vi "flat top.vi"() -> ()   [LabVIEW 2016]
doc: "takes a given beamline component and steps through values and reocrnds the current\noutput from a faraday cup. Allows user to pick highest value"
uses:
  Main/beamline selection.ctl
  Controls/Flat top control settings.ctl
  Controls/flat top states.ctl
  Beamline sections/Main VIs/LowEnd.vi
  Top level/flat top/flat top.lvlib
  Main/main.lvlib
  Beamline sections/Low Energy End/Low energy.lvlib
panel:
  in  "Tab Control":enum32{"Flat Top", "Info", "Errors"}(tab)
  out "Flat top results":cluster{"Y":dbl[], "Y":dbl[]}[](graph)
  in  "Control items":u16(ring) items=["Injector Image X steerer", "Injector Image Y steerer ", "Low Energy Waist  X steerer", "Low Energy Waist Y steerer ", "Tank Entrance  X steerer ", "Tank Entrance Y1 steerer ", "Tank Entrance Y2 steerer ", "Injector Image Einzel ", "Low Energy Einzel ", "Low Energy Waist aperture"]
  in  "Beamline Section":T1
  in  "Flat Top Control Settings":T2={"Start value"=0.0, "Number of steps"=100.0, "Ramp Up Time (s)"=0.0, "End value"=1.0, "Integration Time (s)"=15.0}
  out "step size":dbl
  in  "rare or stable":bool=TRUE
  out "Method of flat top":string
  in  "flat top":bool
  in  "stop":bool
  in  "Help":bool
  out "Main Loop Error":bool=TRUE
  out "Step":i32
  in  "Clear FT Loop Errors":bool
  in  "Clear Main Loop Errors":bool
  out "Main loop error":errorcluster
  out "Flat Top loop error":errorcluster
  out "Original Setting":dbl
  in  "?":cluster{"X":dbl[], "Y":dbl[]}
  in  "error in (no error)":errorcluster
  # "Rare count rate"
  # "Stable Current"
  # "Instructions\n\n1. \n2. \n3."
  # "Notes\n\nPausing/Re-starting\n\nStopping"
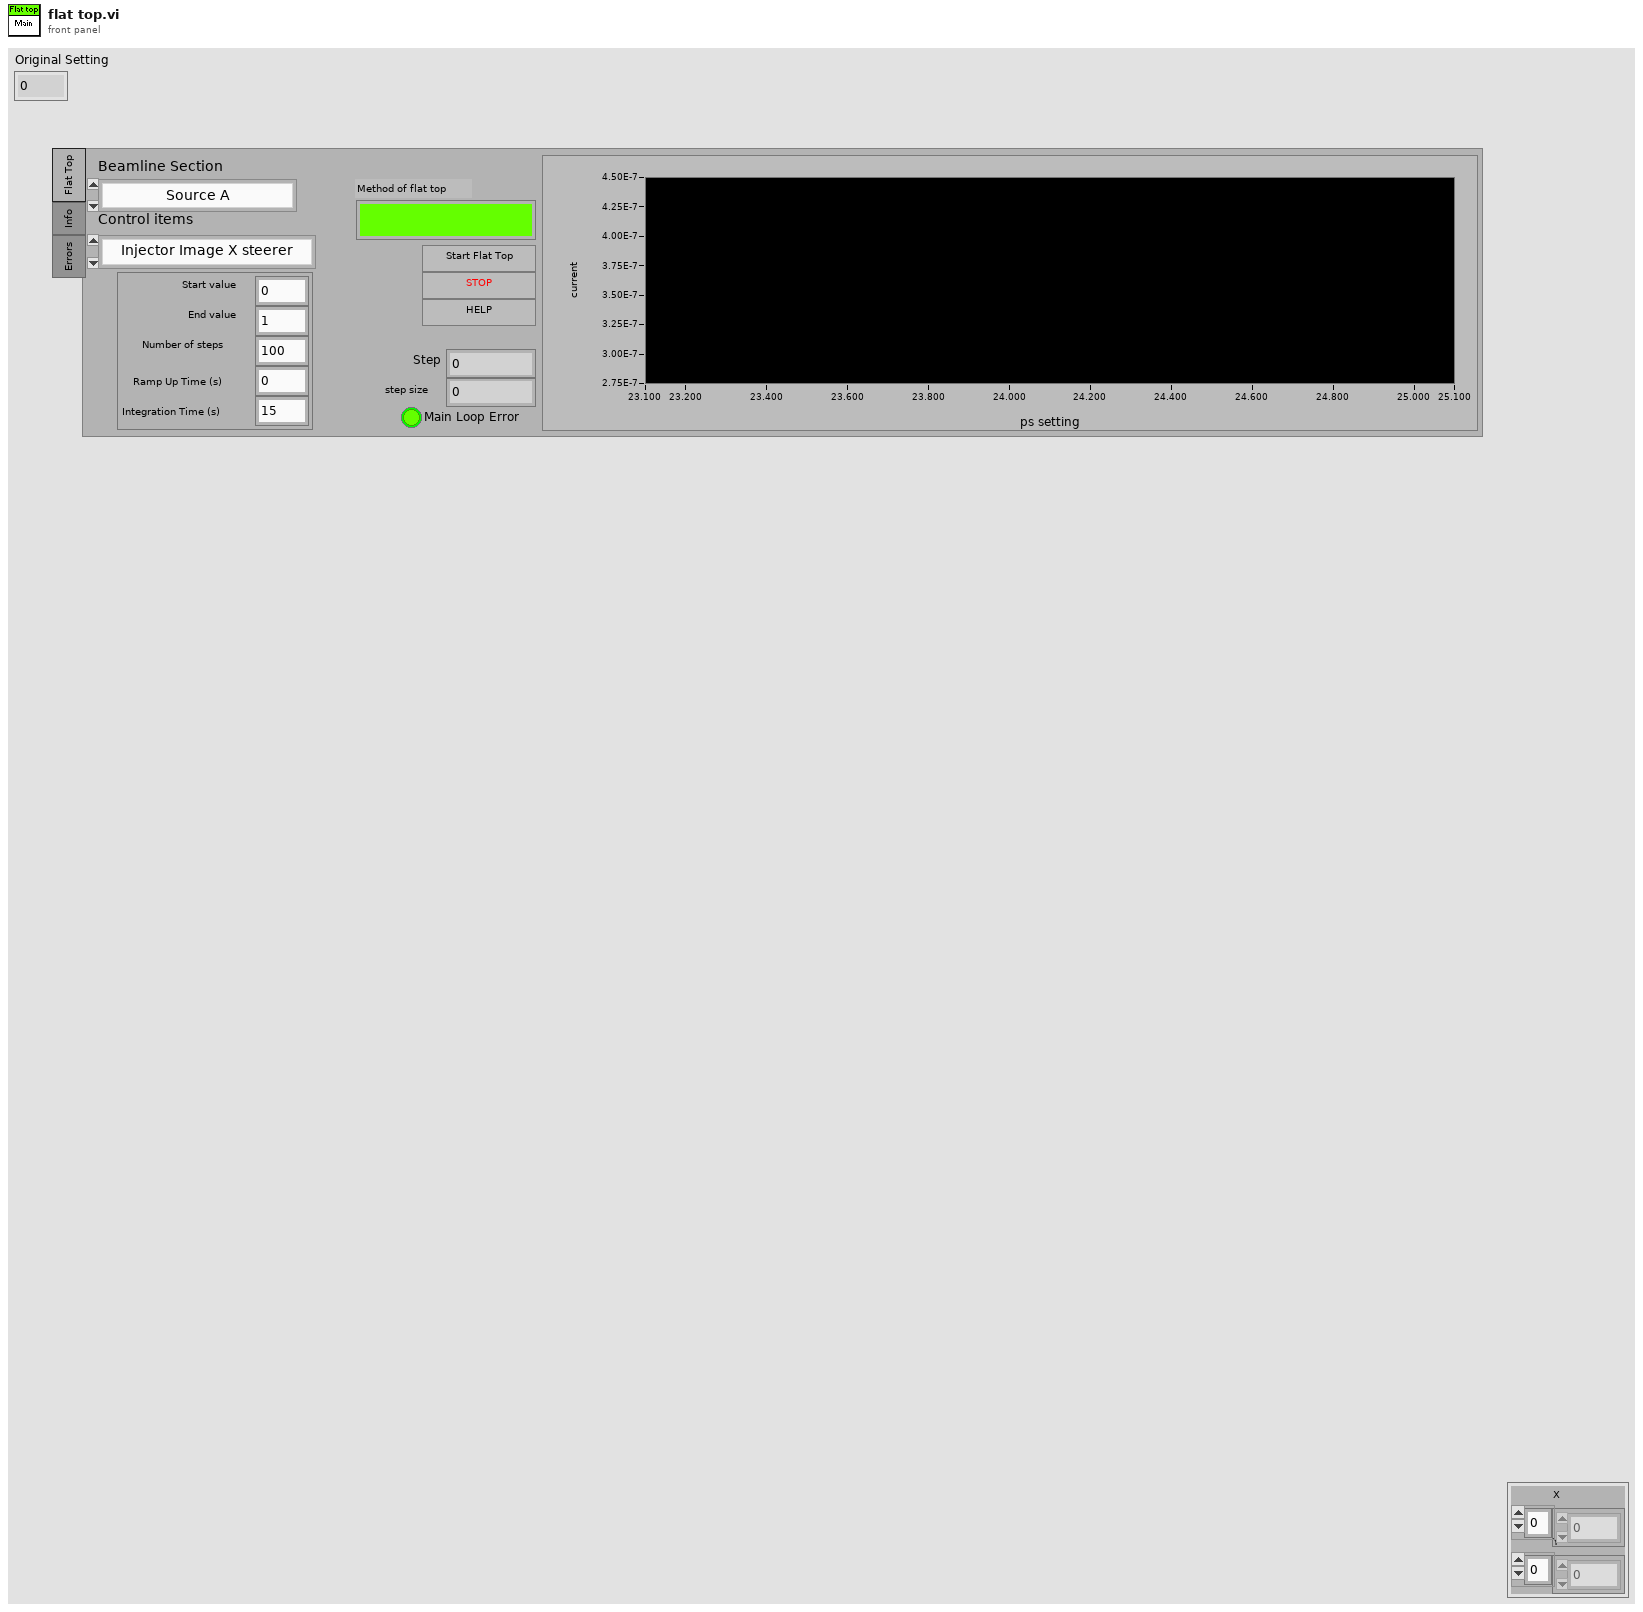
[diagram p1: front panel]
types:
  T1 = typedef "main.lvlib/beamline selection.ctl" = enum16{"Source A", "Low End", "High End", "Transmission", "R30", "R45"}
  T2 = typedef "Flat top control settings.ctl" = cluster{"Start value":dbl, "Number of steps":dbl, "Ramp Up Time (s)":dbl, "End value":dbl, "Integration Time (s)":dbl}
  T3 = typedef "flat top states.ctl" = enum16{"wait", "pause", "flat top", "stop"}
  T4 = cluster{"beamline name":string, "inital value":dbl}[]
  T5 = enum8{"Enabled", "Disabled", "Disabled and Grayed Out"}
  T6 = cluster{"beamline name":string, "inital value":dbl}
  T7 = typedef "LVPoint32TypeDef.ctl" = cluster{"Horizontal":i32, "Vertical":i32}
  T8 = enum16{"Left Button", "Center Button", "Right Button", "Window Close"}
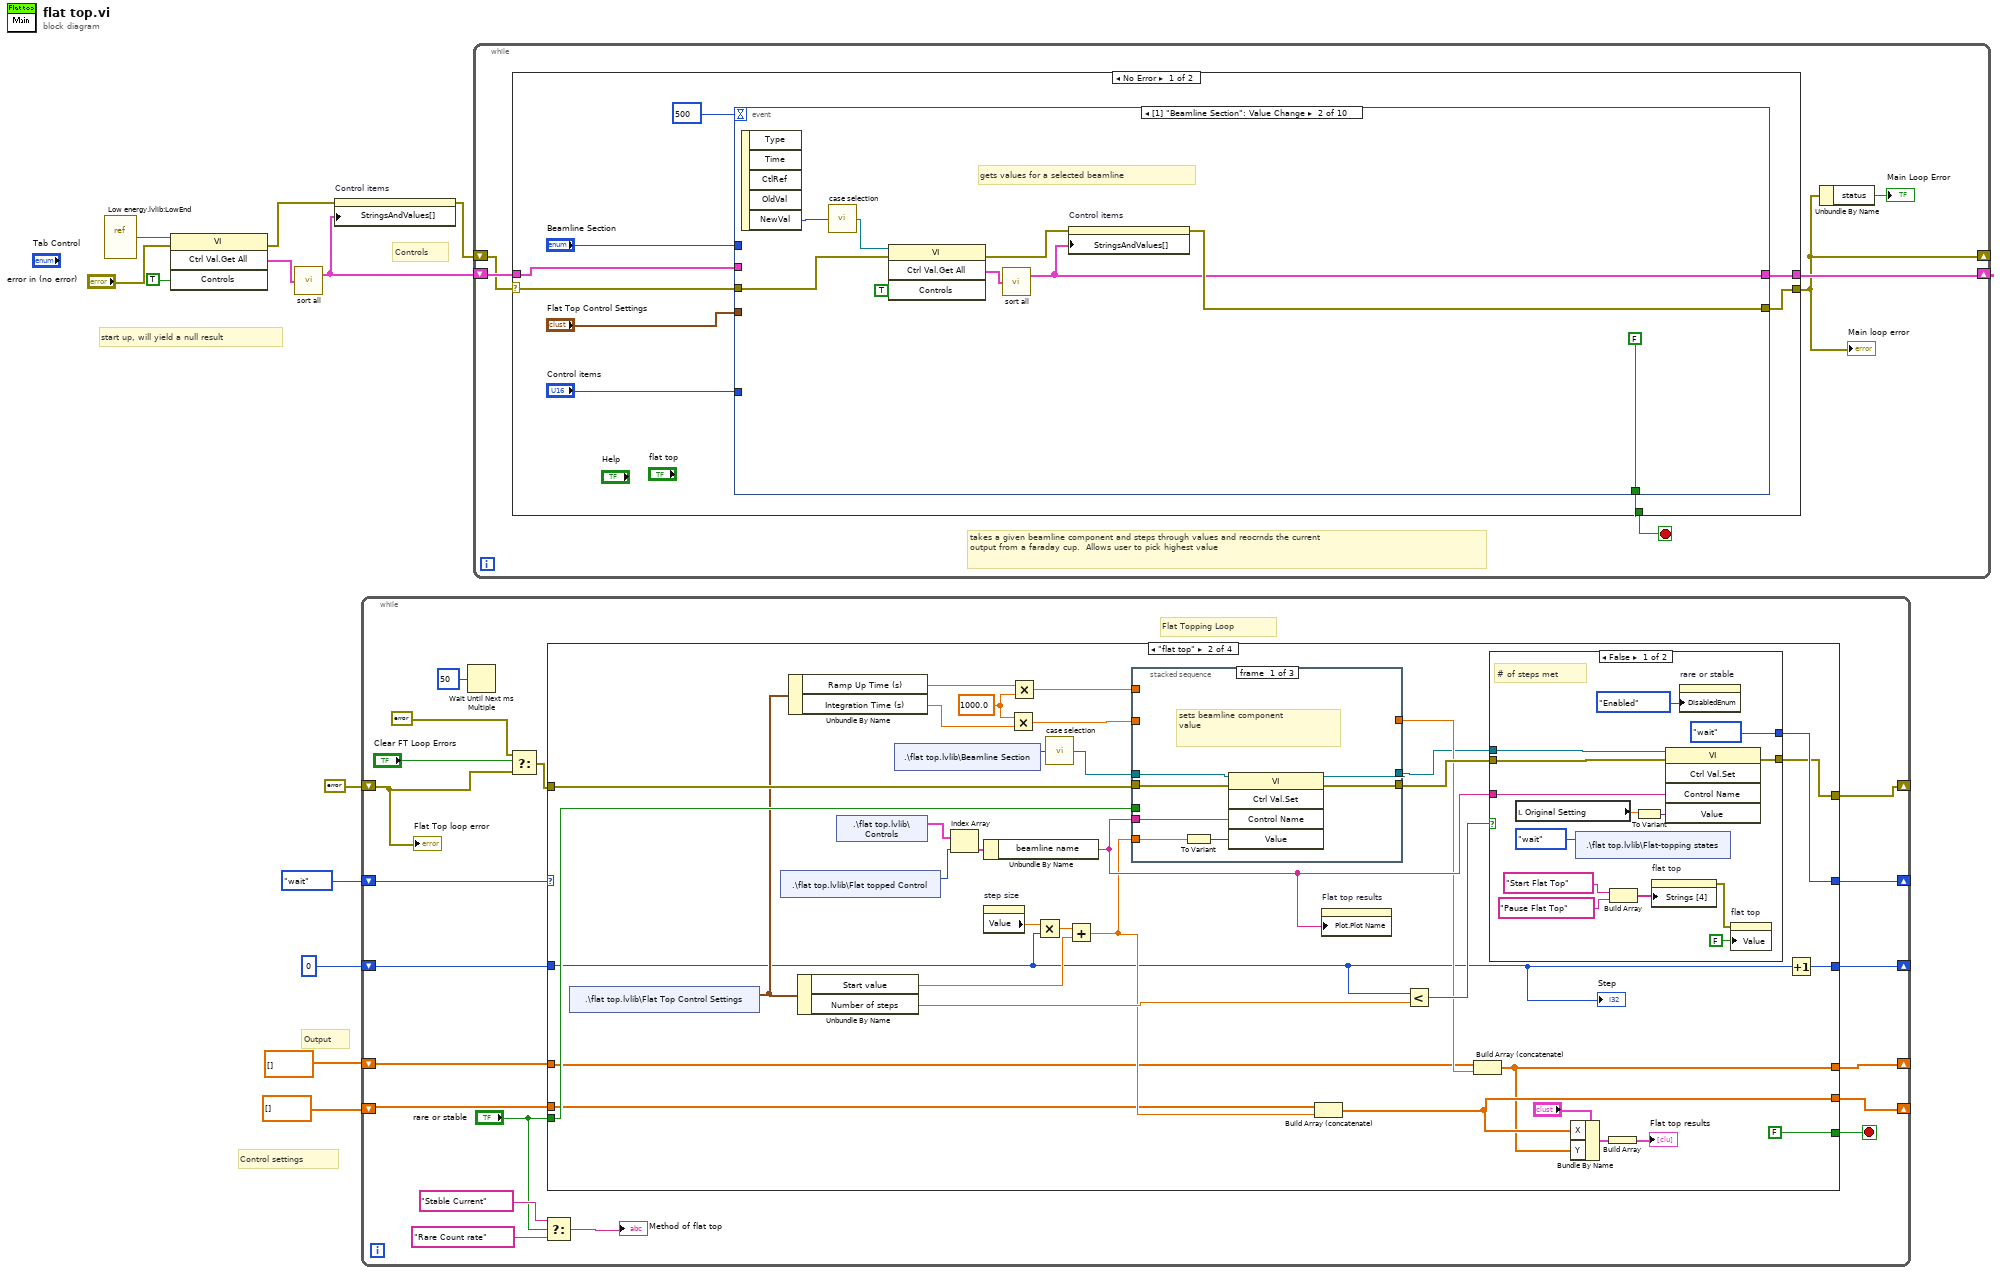
[diagram p0: block diagram]
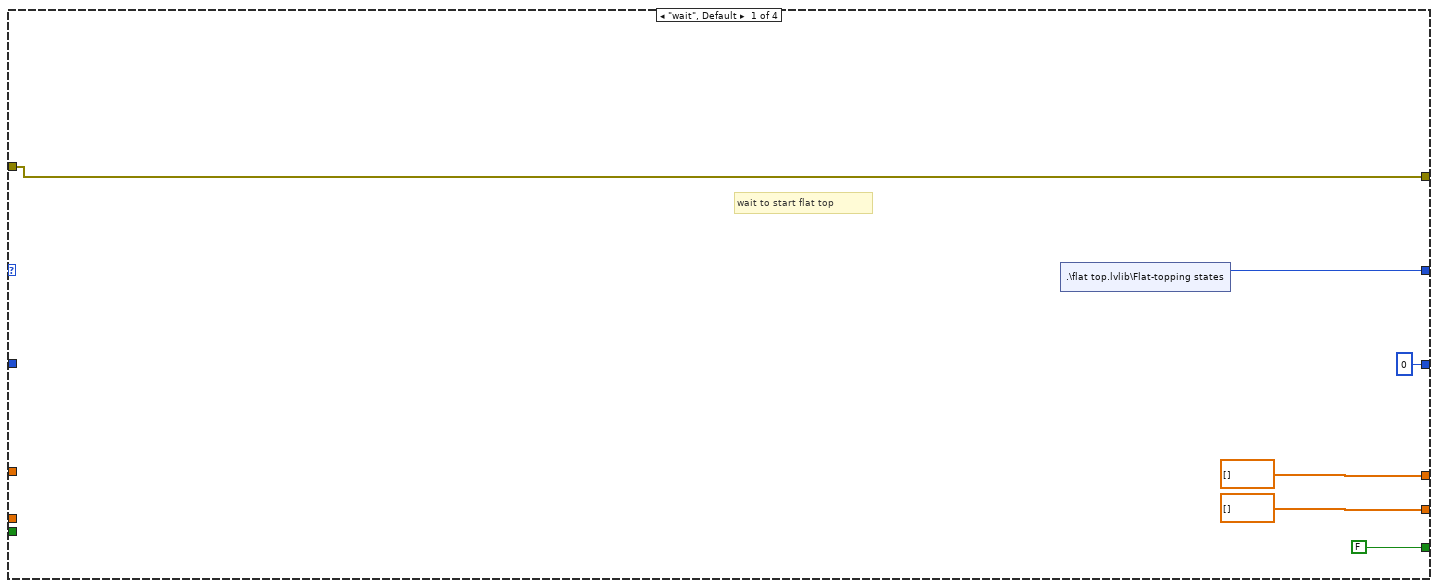
[diagram p2: hidden frame]
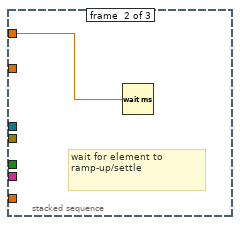
[diagram p3: hidden frame]
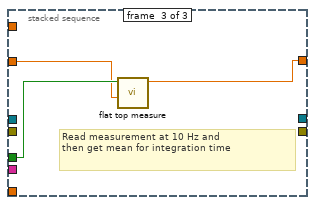
[diagram p4: hidden frame]
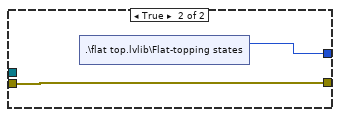
[diagram p5: hidden frame]
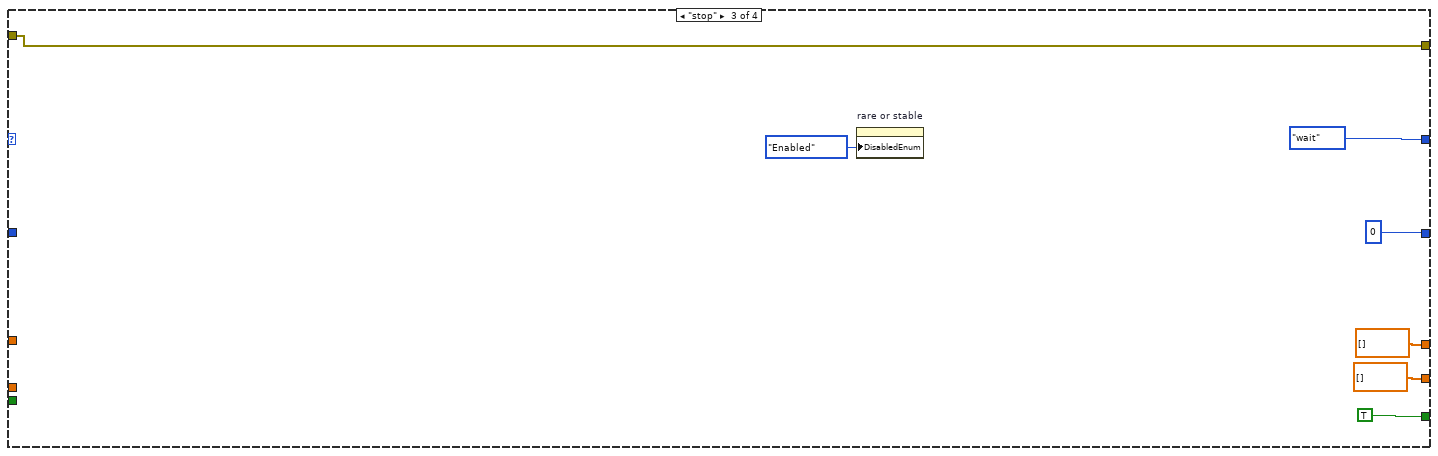
[diagram p6: hidden frame]
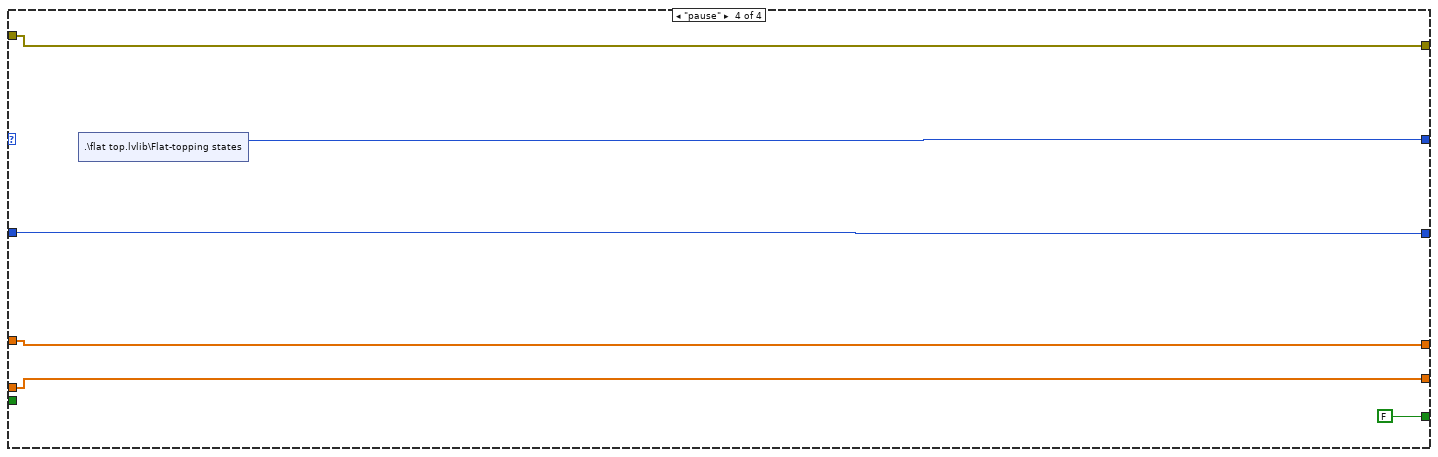
[diagram p7: hidden frame]
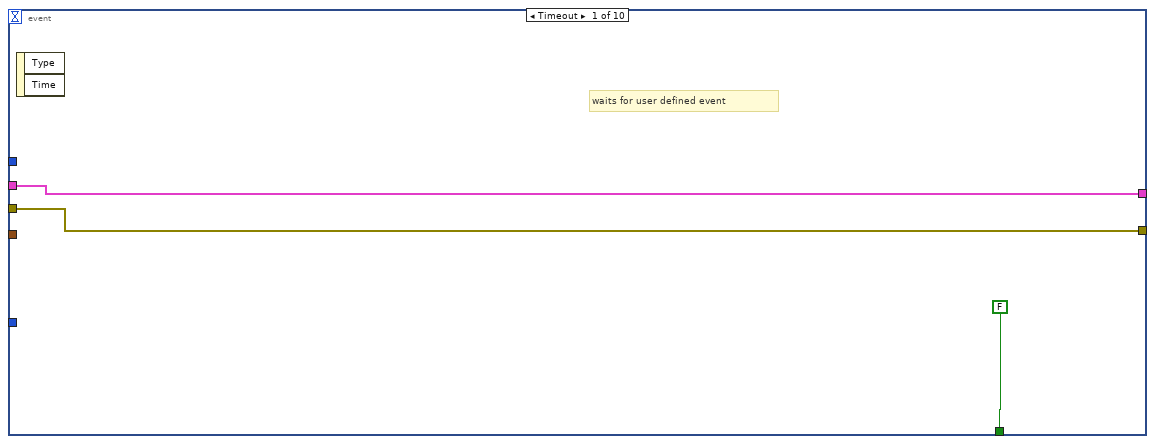
[diagram p8: hidden frame]
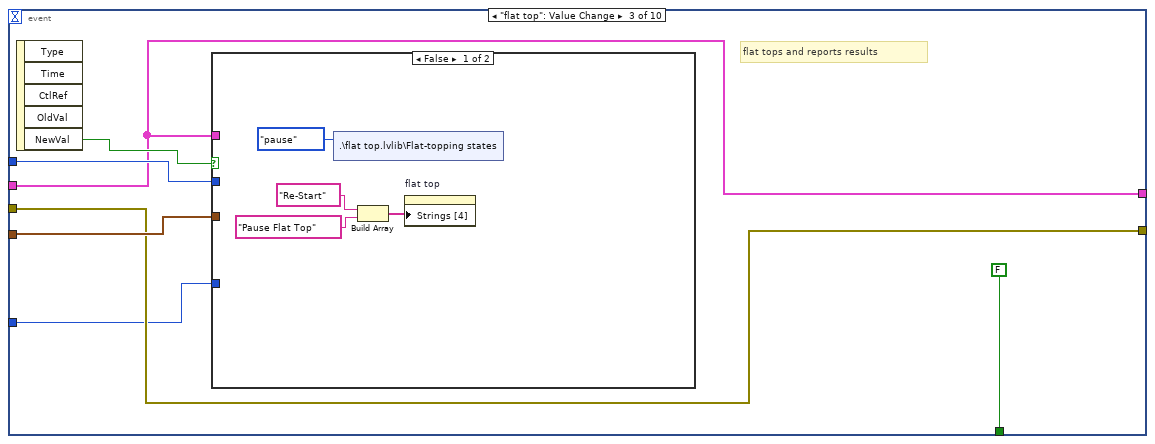
[diagram p9: hidden frame]
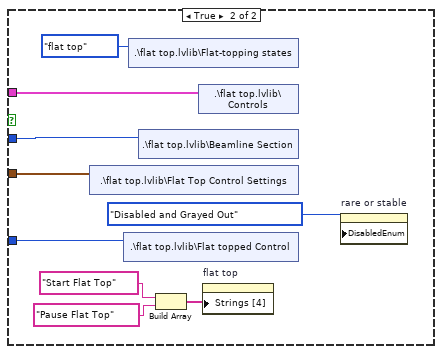
[diagram p10: hidden frame]
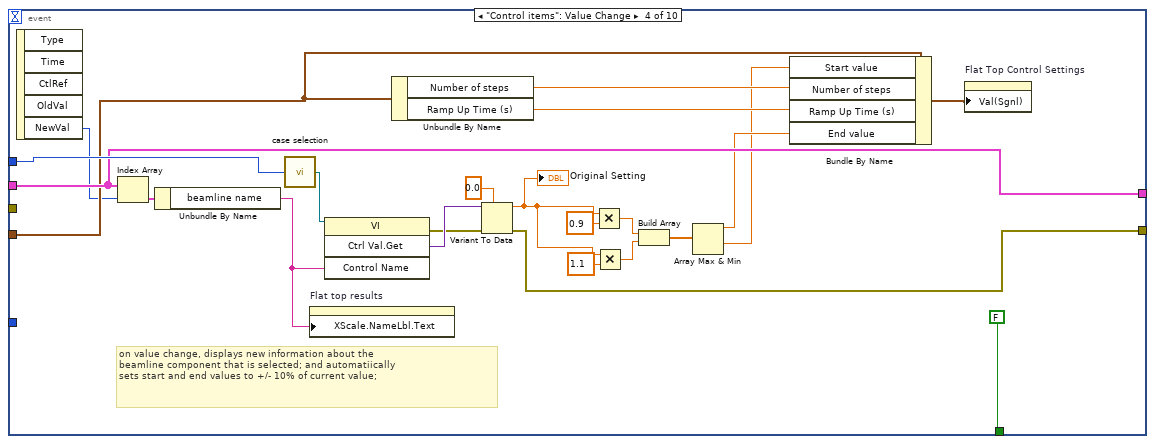
[diagram p11: hidden frame]
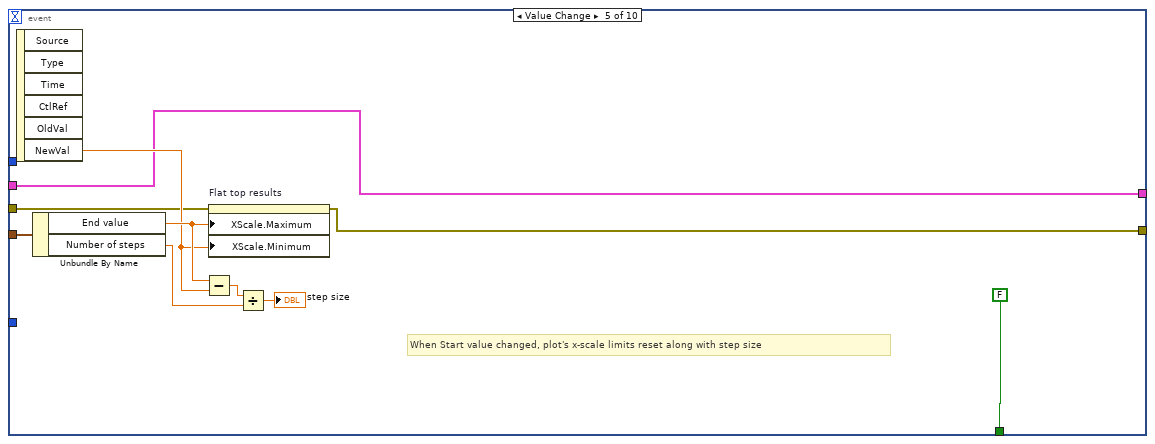
[diagram p12: hidden frame]
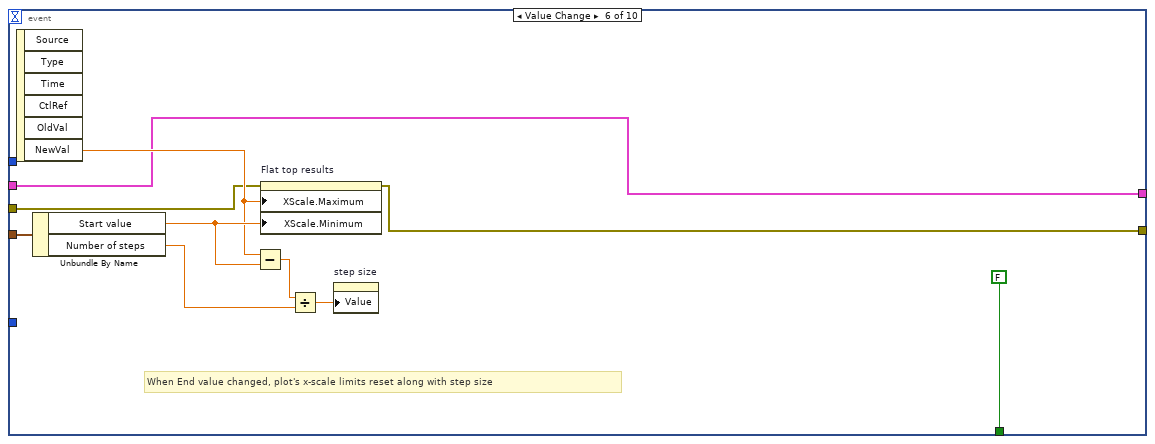
[diagram p13: hidden frame]
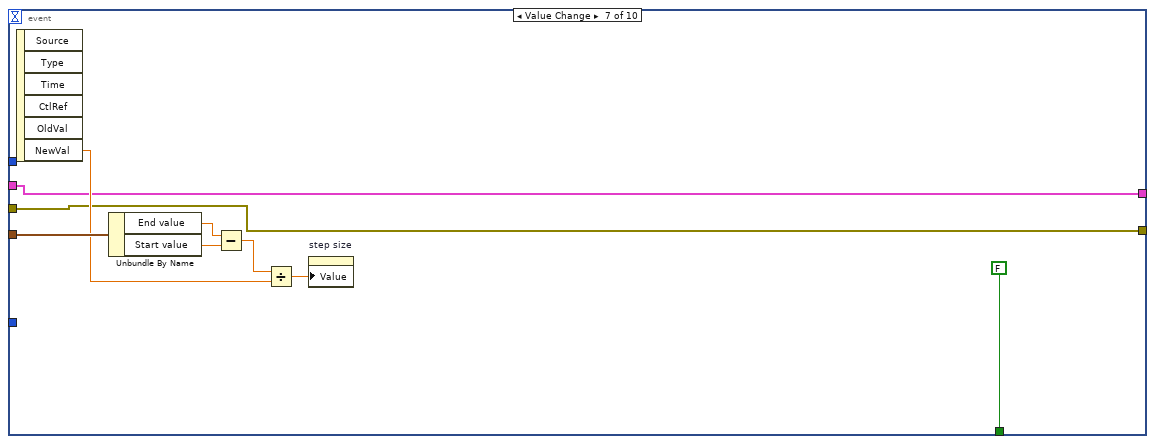
[diagram p14: hidden frame]
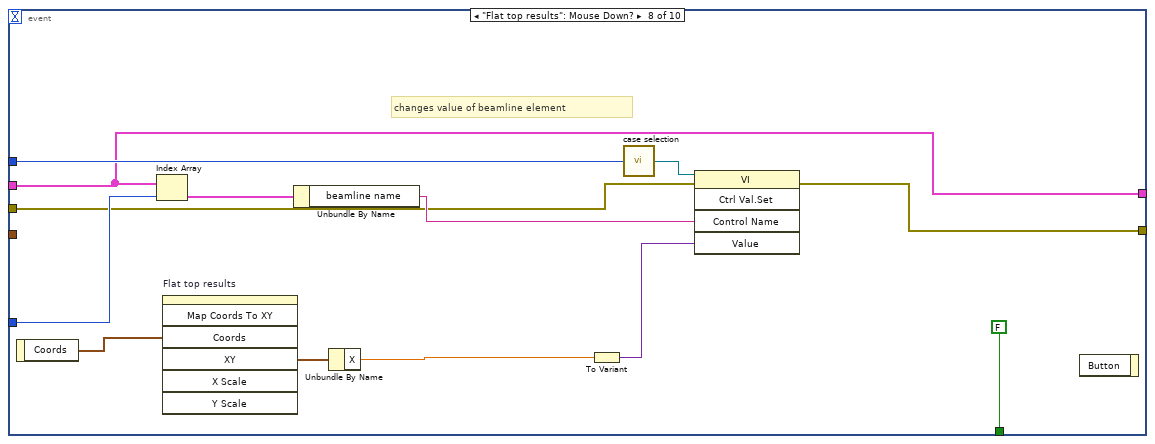
[diagram p15: hidden frame]
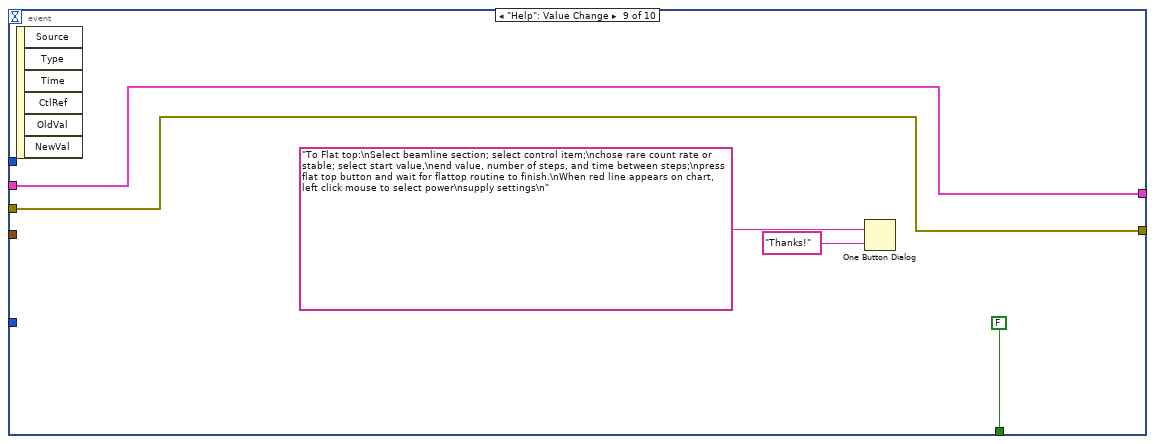
[diagram p16: hidden frame]
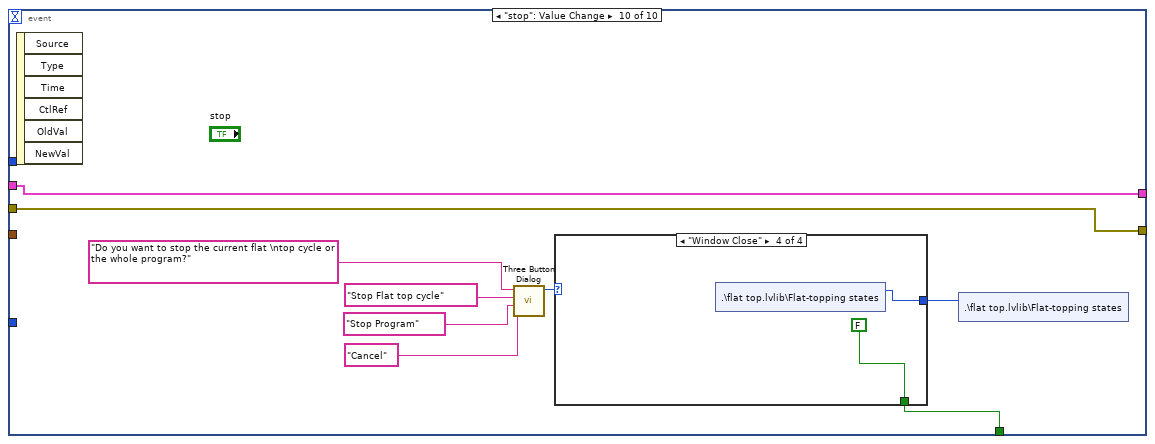
[diagram p17: hidden frame]
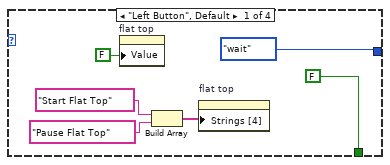
[diagram p18: hidden frame]
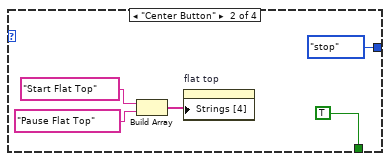
[diagram p19: hidden frame]
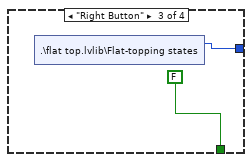
[diagram p20: hidden frame]
diagram:
  # "Control settings"
  # "Output"
  # "Controls"
  # "start up, will yield a null result"
  n1 = vi-ref "Low energy.lvlib:LowEnd.vi"() -> (w8:refnum<vi>)
  n2 = invoke class="VI" method="Ctrl Val.Get All"(reference=w8, error in="error in (no error)", "Controls"=TRUE) -> (error out=w10:errorcluster, "Get All Control Values Variant"=w11:cluster{"Name":string, "Variant Data":variant}[])  [unwired: 1 in, 2 out]
  n3 = call "sort all.vi"("Get All Control Values Variant"=w11) -> ("output"=w9:T4)  [unwired: 1 out]
  n4 = property on="Control items" class="Ring (strict)"(error in=w10, "StringsAndValues[]"=w9) -> (error out=w2:errorcluster)  [unwired: 1 in, 1 out]
  n5 = while {
    shift-right: [w30] -> _
    shift-left: flat_top_states."wait" ("Flat-topping states") -> [w31]
    shift-right: [w25] -> _
    shift-left: 0 -> [w26]
    shift-right: [w23] -> _
    shift-left: dbl[] [] -> [w21]
    shift-right: [w22] -> _
    shift-left: dbl[] [] -> [w20]
    shift-right: [w17] -> _
    shift-left: errorcluster {"status"=FALSE, "code"=0, "source"=""} ("error out") -> [w14]
    stop <- w18 stop-if-true
    # "Flat Topping Loop"
    n6 = Wait Until Next ms Multiple(millisecond multiple=u32 50) -> ()  [unwired: 1 out]
    n7 = Select(t=errorcluster {"status"=FALSE, "code"=0, "source"=""} ("error out"), s="Clear FT Loop Errors", f=w14) -> (s? t:f=w15:errorcluster)
    n8 = Select(t="Stable Current" ("which method of flat top  2"), s="rare or stable", f="Rare Count rate" ("which method of flat top  2")) -> (s? t:f=→"Method of flat top":string)
    n9 = case shown="\"flat top\"" w31 {
      tunnel: [w37 w65 flat_top_states."wait" ("Flat-topping states") w109] -> w30
      tunnel: w26 -> [_ w39 _ w112]
      tunnel: [0 w38 0 w112] -> w25
      tunnel: w15 -> [w33 w58 w101 w107]
      tunnel: "rare or stable" -> [_ w57 _ _]
      tunnel: [dbl[] [] w48 dbl[] [] w111] -> w23
      tunnel: [dbl[] [] w49 dbl[] [] w110] -> w22
      tunnel: w21 -> [_ w51 _ w111]
      tunnel: w20 -> [_ w50 _ w110]
      tunnel: [FALSE FALSE TRUE FALSE] -> w18
      tunnel: [w33 w46 w101 w107] -> w17
      frame "wait", Default {
        # "wait to start flat top"
        n10 = shared-variable ".\\flat top.lvlib\\Flat-topping states"() -> (w37:T3)  [unwired: 1 in, 1 out]
      }
      frame "flat top" {
        w42 = 1000.0 ("y")
        n11 = shared-variable ".\\flat top.lvlib\\Flat Top Control Settings"() -> (w45:T2)  [unwired: 1 in, 1 out]
        n12 = shared-variable ".\\flat top.lvlib\\Flat topped Control"() -> (w70:u16)  [unwired: 1 in, 1 out]
        n13 = Unbundle By Name(w45) -> ("Ramp Up Time (s)"=w43:dbl, "Integration Time (s)"=w44:dbl)
        n14 = Unbundle By Name(w45) -> ("Start value"=w60:dbl, "Number of steps"=w63:dbl)
        n15 = shared-variable ".\\flat top.lvlib\\Controls"() -> (w71:T4)  [unwired: 1 in, 1 out]
        n16 = shared-variable ".\\flat top.lvlib\\Beamline Section"() -> (w72:T1)  [unwired: 1 in, 1 out]
        n17 = Index Array(array=w71, index=w70) -> (element=w69:T6)
        n18 = Unbundle By Name(w69) -> ("beamline name"=w55:string)
        n19 = property on="step size" class="DigNum (strict)"() -> ("Value"=w61:dbl)  [unwired: 2 in, 2 out]
        n20 = Multiply(x=w42, y=w44) -> (x*y=w54:dbl)
        n21 = Multiply(x=w43, y=w42) -> (x*y=w41:dbl)
        n22 = Multiply(x=w61, y=w39) -> (x*y=w62:dbl)
        n23 = call "case selection.vi"("Beamline Section"=w72) -> ("VI Refnum"=w59:refnum<vi>)
        n24 = Add(x=w62, y=w60) -> (x+y=w53:dbl)
        n25 = stacked-sequence {
          tunnel: w59 -> [w78 _ _]
          tunnel: w58 -> [w77 _ _]
          tunnel: w55 -> [w76 _ _]
          tunnel: w53 -> [w75 _ _]
          tunnel: [_ _ w83] -> w52
          tunnel: [w73 _ _] -> w56
          tunnel: w54 -> [_ _ w81]
          tunnel: w57 -> [_ _ w82]
          tunnel: w41 -> [_ w80 _]
          tunnel: [w74 _ _] -> w40
          frame #0 {
            # "sets beamline component \nvalue"
            n26 = To Variant(anything=w75) -> (Variant=w79:variant)
            n27 = invoke class="VI" method="Ctrl Val.Set"(reference=w78, error in=w77, "Control Name"=w76, "Value"=w79) -> (reference out=w74:refnum<vi>, error out=w73:errorcluster)  [unwired: 1 in, 3 out]
          }
          frame #1 {
            # "wait for element to \nramp-up/settle"
            n28 = Wait (ms)(milliseconds to wait=w80) -> ()  [unwired: 1 out]
          }
          frame #2 {
            # "Read measurement at 10 Hz and \nthen get mean for integration time"
            n29 = call "flat top measure.vi"("Integration time"=w81, "rare or stable"=w82) -> ("Measurement"=w83:dbl)  [unwired: 9 in]
          }
        }
        n30 = Build Array (concatenate)(w50, w53) -> (w49:dbl[])
        n31 = property on="Flat top results" class="XYGraph (strict)"("Plot.Plot Name"=w55) -> ()  [unwired: 2 in, 2 out]
        n32 = Less?(x=w39, y=w63) -> (x < y?=w64:bool)
        n33 = Build Array (concatenate)(w51, w52) -> (w48:dbl[])
        n34 = case shown="False" w64 {
          tunnel: [flat_top_states."wait" ("Flat-topping states") w99] -> w65
          tunnel: w40 -> [w96 _]
          tunnel: w55 -> [w95 _]
          tunnel: w56 -> [w92 w98]
          tunnel: [w91 w98] -> w46
          frame False {
            # "# of steps met"
            n35 = local read "Original Setting"() -> (w93:dbl)
            n36 = shared-variable ".\\flat top.lvlib\\Flat-topping states"(flat_top_states."wait" ("Flat-topping states")) -> ()  [unwired: 1 in, 1 out]
            n37 = Build Array("Start Flat Top" ("Boolean Text.Text"), "Pause Flat Top" ("element")) -> (w86:string[])
            n38 = To Variant(anything=w93) -> (Variant=w94:variant)
            n39 = property on="flat top" class="Bool (strict)"("Strings [4]"=w86) -> (error out=w84:errorcluster)  [unwired: 2 in, 1 out]
            n40 = invoke class="VI" method="Ctrl Val.Set"(reference=w96, error in=w92, "Control Name"=w95, "Value"=w94) -> (error out=w91:errorcluster)  [unwired: 1 in, 4 out]
            n41 = property on="rare or stable" class="Bool (strict)"("DisabledEnum"=T5."Enabled" ("Disabled")) -> ()  [unwired: 2 in, 2 out]
            n42 = property on="flat top" class="Bool (strict)"(error in=w84, "Value"=FALSE ("flat top")) -> ()  [unwired: 1 in, 2 out]
          }
          frame True {
            n43 = shared-variable ".\\flat top.lvlib\\Flat-topping states"() -> (w99:T3)  [unwired: 1 in, 1 out]
          }
        }
        n44 = Bundle By Name(cluster="?", "X"=w49, "Y"=w48) -> (w67:cluster{"X":dbl[], "Y":dbl[]})
        n45 = Build Array(w67) -> (→"Flat top results":cluster{"X":dbl[], "Y":dbl[]}[])
        n46 = Increment(x=w39) -> (x+1=w38:i32)
        "Step" <- w39
      }
      frame "stop" {
        n47 = property on="rare or stable" class="Bool (strict)"("DisabledEnum"=T5."Enabled" ("Disabled")) -> ()  [unwired: 2 in, 2 out]
      }
      frame "pause" {
        n48 = shared-variable ".\\flat top.lvlib\\Flat-topping states"() -> (w109:T3)  [unwired: 1 in, 1 out]
      }
    }
    "Flat Top loop error" <- w14
  }
  n49 = while {
    shift-right: [w118] -> _
    shift-left: w9 -> [w117]
    shift-right: [w114] -> _
    shift-left: w2 -> [w115]
    stop <- w116 stop-if-true
    # "takes a given beamline component and steps through values and reocrnds the current\noutput from a faraday cup.  Allows user to pick highest value"
    n50 = case shown="No Error" w115 {
      selector: w115 -> [w121 w255]
      tunnel: [w126 w257] -> w118
      tunnel: w117 -> [w125 w257]
      tunnel: [w123 w254] -> w114
      tunnel: [w119 FALSE ("stop")] -> w116
      frame No Error {
        n51 = event shown="[1] \"Beamline Section\": Value Change" {
          selector: _ -> [_ _ _ _ _ _ _ _ _ _]
          dyn-events: _ -> [_ _ _ _ _ _ _ _ _ _]
          timeout: 500 -> [_ _ _ _ _ _ _ _ _ _]
          tunnel: [w130 w134 w141 w176 w186 w194 w204 w213 w226 w237] -> w126
          tunnel: w125 -> [w130 _ w141 w176 w186 w194 w204 w213 w226 w237]
          tunnel: w121 -> [w129 w136 w143 _ w185 w196 w205 w216 w227 w238]
          tunnel: "Control items" -> [_ _ w140 _ _ _ _ w220 _ _]
          tunnel: [w129 w139 w143 w161 w184 w195 w205 w215 w227 w238] -> w123
          tunnel: "Beamline Section" -> [_ _ w145 w177 _ _ _ w218 _ _]
          tunnel: "Flat Top Control Settings" -> [_ _ w144 w172 w188 w199 w208 _ _ _]
          tunnel: [FALSE ("stop") FALSE ("stop") FALSE ("stop") FALSE ("stop") FALSE ("stop") FALSE ("stop") FALSE ("stop") FALSE ("stop") FALSE ("stop") w231] -> w119
          event Timeout {
            # "waits for user defined event"
            n52 = event-data() -> ()  [unwired: 1 in, 2 out]
          }
          event Value Change {
            # "gets values for a selected beamline"
            n53 = event-data() -> ("NewVal"=w138:T1)  [unwired: 1 in, 4 out]
            n54 = call "case selection.vi"("Beamline Section"=w138) -> ("VI Refnum"=w135:refnum<vi>)
            n55 = invoke class="VI" method="Ctrl Val.Get All"(reference=w135, error in=w136, "Controls"=TRUE) -> (error out=w137:errorcluster, "Get All Control Values Variant"=w132:cluster{"Name":string, "Variant Data":variant}[])  [unwired: 1 in, 2 out]
            n56 = call "sort all.vi"("Get All Control Values Variant"=w132) -> ("output"=w134:T4)  [unwired: 1 out]
            n57 = property on="Control items" class="Ring (strict)"(error in=w137, "StringsAndValues[]"=w134) -> (error out=w139:errorcluster)  [unwired: 1 in, 1 out]
          }
          event "flat top": Value Change {
            # "flat tops and reports results"
            n58 = event-data() -> ("NewVal"=w146:bool)  [unwired: 1 in, 4 out]
            n59 = case shown="False" w146 {
              tunnel: w140 -> [_ w158]
              tunnel: w145 -> [_ w157]
              tunnel: w144 -> [_ w156]
              tunnel: w141 -> [_ w155]
              frame False {
                n60 = shared-variable ".\\flat top.lvlib\\Flat-topping states"(flat_top_states."pause" ("Flat-topping states")) -> ()  [unwired: 1 in, 1 out]
                n61 = Build Array("Re-Start" ("Boolean Text.Text"), "Pause Flat Top" ("element")) -> (w147:string[])
                n62 = property on="flat top" class="Bool (strict)"("Strings [4]"=w147) -> ()  [unwired: 2 in, 2 out]
              }
              frame True {
                n63 = shared-variable ".\\flat top.lvlib\\Flat Top Control Settings"(w156) -> ()  [unwired: 1 in, 1 out]
                n64 = shared-variable ".\\flat top.lvlib\\Flat topped Control"(w158) -> ()  [unwired: 1 in, 1 out]
                n65 = shared-variable ".\\flat top.lvlib\\Flat-topping states"(flat_top_states."flat top" ("Flat-topping states")) -> ()  [unwired: 1 in, 1 out]
                n66 = shared-variable ".\\flat top.lvlib\\Beamline Section"(w157) -> ()  [unwired: 1 in, 1 out]
                n67 = Build Array("Start Flat Top" ("Boolean Text.Text"), "Pause Flat Top" ("element")) -> (w152:string[])
                n68 = shared-variable ".\\flat top.lvlib\\Controls"(w155) -> ()  [unwired: 1 in, 1 out]
                n69 = property on="flat top" class="Bool (strict)"("Strings [4]"=w152) -> ()  [unwired: 2 in, 2 out]
                n70 = property on="rare or stable" class="Bool (strict)"("DisabledEnum"=T5."Disabled and Grayed Out" ("Disabled")) -> ()  [unwired: 2 in, 2 out]
              }
            }
          }
          event "Control items": Value Change {
            # "on value change, displays new information about the \nbeamline component that is selected; and automatiically\nsets start and end values to +/- 10% of current value;"
            n71 = event-data() -> ("NewVal"=w163:u16)  [unwired: 1 in, 4 out]
            n72 = Index Array(array=w176, index=w163) -> (element=w182:T6)
            n73 = Unbundle By Name(w182) -> ("beamline name"=w162:string)
            n74 = call "case selection.vi"("Beamline Section"=w177) -> ("VI Refnum"=w178:refnum<vi>)
            n75 = property on="Flat top results" class="XYGraph (strict)"("XScale.NameLbl.Text"=w162) -> ()  [unwired: 2 in, 2 out]
            n76 = invoke class="VI" method="Ctrl Val.Get"(reference=w178, "Control Name"=w162) -> (error out=w180:errorcluster, "Get Control Value Variant"=w181:variant)  [unwired: 2 in, 2 out]
            n77 = Unbundle By Name(w172) -> ("Number of steps"=w175:dbl, "Ramp Up Time (s)"=w174:dbl)
            n78 = Variant To Data(error in=w180, type=0.0, Variant=w181) -> (data=w169:dbl, error out=w161:errorcluster)
            "Original Setting" <- w169
            n79 = Multiply(x=w169, y=0.9) -> (x*y=w167:dbl)
            n80 = Multiply(x=w169, y=1.1) -> (x*y=w168:dbl)
            n81 = Build Array(w167, w168) -> (w166:dbl[])
            n82 = Array Max & Min(array=w166) -> (max value=w165:dbl, min value=w164:dbl)  [unwired: 2 out]
            n83 = Bundle By Name(cluster=w172, "Start value"=w164, "Number of steps"=w175, "Ramp Up Time (s)"=w174, "End value"=w165) -> (w173:T2)
            n84 = property on="Flat Top Control Settings" class="Clust (strict)"("Val(Sgnl)"=w173) -> ()  [unwired: 2 in, 2 out]
          }
          event Value Change {
            # "When Start value changed, plot's x-scale limits reset along with step size"
            n85 = event-data() -> ("NewVal"=w187:dbl)  [unwired: 1 in, 5 out]
            n86 = Unbundle By Name(w188) -> ("End value"=w190:dbl, "Number of steps"=w191:dbl)
            n87 = Subtract(x=w190, y=w187) -> (x-y=w189:dbl)
            n88 = property on="Flat top results" class="XYGraph (strict)"(error in=w185, "XScale.Maximum"=w190, "XScale.Minimum"=w187) -> (error out=w184:errorcluster)  [unwired: 1 in, 1 out]
            n89 = Divide(x=w189, y=w191) -> (x/y=→"step size":dbl)
          }
          event Value Change {
            # "When End value changed, plot's x-scale limits reset along with step size"
            n90 = event-data() -> ("NewVal"=w198:dbl)  [unwired: 1 in, 5 out]
            n91 = Unbundle By Name(w199) -> ("Start value"=w201:dbl, "Number of steps"=w202:dbl)
            n92 = Subtract(x=w198, y=w201) -> (x-y=w200:dbl)
            n93 = property on="Flat top results" class="XYGraph (strict)"(error in=w196, "XScale.Maximum"=w198, "XScale.Minimum"=w201) -> (error out=w195:errorcluster)  [unwired: 1 in, 1 out]
            n94 = Divide(x=w200, y=w202) -> (x/y=w197:dbl)
            n95 = property on="step size" class="DigNum (strict)"("Value"=w197) -> ()  [unwired: 2 in, 2 out]
          }
          event Value Change {
            n96 = event-data() -> ("NewVal"=w207:dbl)  [unwired: 1 in, 5 out]
            n97 = Unbundle By Name(w208) -> ("End value"=w210:dbl, "Start value"=w211:dbl)
            n98 = Subtract(x=w210, y=w211) -> (x-y=w209:dbl)
            n99 = Divide(x=w209, y=w207) -> (x/y=w206:dbl)
            n100 = property on="step size" class="DigNum (strict)"("Value"=w206) -> ()  [unwired: 2 in, 2 out]
          }
          event "Flat top results": Mouse Down? {
            # "changes value of beamline element"
            n101 = event-data() -> ("Coords"=w224:T7)  [unwired: 1 in]
            n102 = Index Array(array=w213, index=w220) -> (element=w221:T6)
            n103 = invoke on="Flat top results" class="XYGraph (strict)" method="Map Coords To XY"("Coords"=w224) -> ("XY"=w222:cluster{"X":dbl, "Y":dbl})  [unwired: 6 in, 6 out]
            n104 = Unbundle By Name(w221) -> ("beamline name"=w219:string)
            n105 = Unbundle By Name(w222) -> ("X"=w214:dbl)
            n106 = To Variant(anything=w214) -> (Variant=w223:variant)
            n107 = call "case selection.vi"("Beamline Section"=w218) -> ("VI Refnum"=w217:refnum<vi>)
            n108 = invoke class="VI" method="Ctrl Val.Set"(reference=w217, error in=w216, "Control Name"=w219, "Value"=w223) -> (error out=w215:errorcluster)  [unwired: 1 in, 4 out]
            n109 = event-data() -> ()  [unwired: 2 in, 1 out]
          }
          event "Help": Value Change {
            n110 = event-data() -> ()  [unwired: 1 in, 6 out]
            n111 = One Button Dialog(message="To Flat top:\nSelect beamline section; select control item;\nchose rare count rate or stable; select start value,\nend value, number of steps, and time between steps;\npress flat top button and wait for flattop routine to finish.\nWhen red line appears on chart, left click mouse to select power\nsupply settings\n", button name ("OK")="Thanks!") -> ()  [unwired: 1 out]
          }
          event "stop": Value Change {
            n112 = event-data() -> ()  [unwired: 1 in, 6 out]
            n113 = call <vilib>:"Three Button Dialog.vi"("Right Button Text (\"Cancel\")"="Cancel" ("Right Button Text (\"Cancel\")"), "Center Button Text (\"No\")"="Stop Program" ("Center Button Text (\"No\")"), "Left Button Text (\"Yes\")"="Stop Flat top cycle" ("Left Button Text (\"Yes\")"), "message"="Do you want to stop the current flat \ntop cycle or the whole program?") -> ("Which Button?"=w233:T8)  [unwired: 7 in]
            n114 = case shown="\"Window Close\"" w233 {
              tunnel: [flat_top_states."wait" ("Flat-topping states") flat_top_states."stop" ("Flat-topping states") w250 w252] -> w232
              tunnel: [FALSE ("stop") TRUE ("stop") FALSE ("stop") FALSE ("stop")] -> w231
              frame "Left Button", Default {
                n115 = property on="flat top" class="Bool (strict)"("Value"=FALSE ("flat top")) -> ()  [unwired: 2 in, 2 out]
                n116 = Build Array("Start Flat Top" ("Boolean Text.Text"), "Pause Flat Top" ("element")) -> (w240:string[])
                n117 = property on="flat top" class="Bool (strict)"("Strings [4]"=w240) -> ()  [unwired: 2 in, 2 out]
              }
              frame "Center Button" {
                n118 = Build Array("Start Flat Top" ("Boolean Text.Text"), "Pause Flat Top" ("element")) -> (w246:string[])
                n119 = property on="flat top" class="Bool (strict)"("Strings [4]"=w246) -> ()  [unwired: 2 in, 2 out]
              }
              frame "Right Button" {
                n120 = shared-variable ".\\flat top.lvlib\\Flat-topping states"() -> (w250:T3)  [unwired: 1 in, 1 out]
              }
              frame "Window Close" {
                n121 = shared-variable ".\\flat top.lvlib\\Flat-topping states"() -> (w252:T3)  [unwired: 1 in, 1 out]
              }
            }
            n122 = shared-variable ".\\flat top.lvlib\\Flat-topping states"(w232) -> ()  [unwired: 1 in, 1 out]
          }
        }
      }
      frame Error {
        n123 = case shown="True" "Clear Main Loop Errors" {
          tunnel: w255 -> [w259 w261]
          tunnel: [w259 w260] -> w254
          frame False {
          }
          frame True {
            n124 = call <vilib>:"Clear Errors.vi"("error in (no error)"=w261) -> ("error out"=w260:errorcluster)  [unwired: 5 in, 1 out]
          }
        }
      }
    }
    "Main loop error" <- w114
    n125 = Unbundle By Name(w114) -> ("status"=→"Main Loop Error":bool)
  }
